vi "Parse RMC Sentence.vi"(8 "error in (no error)":errorcluster, 11 "RMC sentence":string) -> (0 "error out":errorcluster, 3 "RMC data":T1 {"type of fix"."mode" items=["Simulator", "Not Valid", "Estimated", "Differential", "Autonomous"]; "status"."value" items=["Void", "Active"]; "time of fix"."time (UTC)" format=" %^<%.3X\n%x>T"})   [LabVIEW 2017, in "NMEA API.lvlib"]
doc: "Returns data contained in a particular type of NMEA sentence. The input sentence you specify must include valid NMEA formatting and end with a carriage return and line feed, or \\r\\n. You must manually select the polymorphic instance to use."
uses:
  <vilib>/robotics/Protocols/NMEA/NMEA API.lvlib
  <vilib>/robotics/Protocols/NMEA/typedefs/RMC Data.ctl
  <vilib>/Utility/miscctls.llb/LVDateTimeRec.ctl
  <vilib>/robotics/Utilities/NI_Robotics Utilities.lvlib
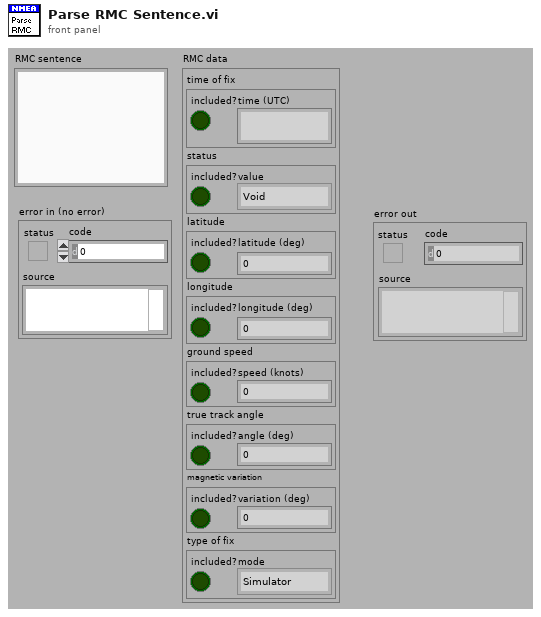
[diagram p1: front panel]
types:
  T1 = typedef "NMEA API.lvlib/RMC Data.ctl" = cluster{"time of fix":cluster{"included?":bool, "time (UTC)":timestamp}, "status":cluster{"included?":bool, "value":u16}, "latitude":cluster{"included?":bool, "latitude (deg)":dbl}, "longitude":cluster{"included?":bool, "longitude (deg)":dbl}, "ground speed":cluster{"included?":bool, "speed (knots)":dbl}, "true track angle":cluster{"included?":bool, "angle (deg)":dbl}, "magnetic variation":cluster{"included?":bool, "variation (deg)":dbl}, "type of fix":cluster{"included?":bool, "mode":u16}}
  T2 = typedef "LVDateTimeRec.ctl" = cluster{"fractional second":dbl, "second":i32, "minute":i32, "hour":i32, "day of month":i32, "month":i32, "year":i32, "day of week":i32, "day of year":i32, "DST":i32}
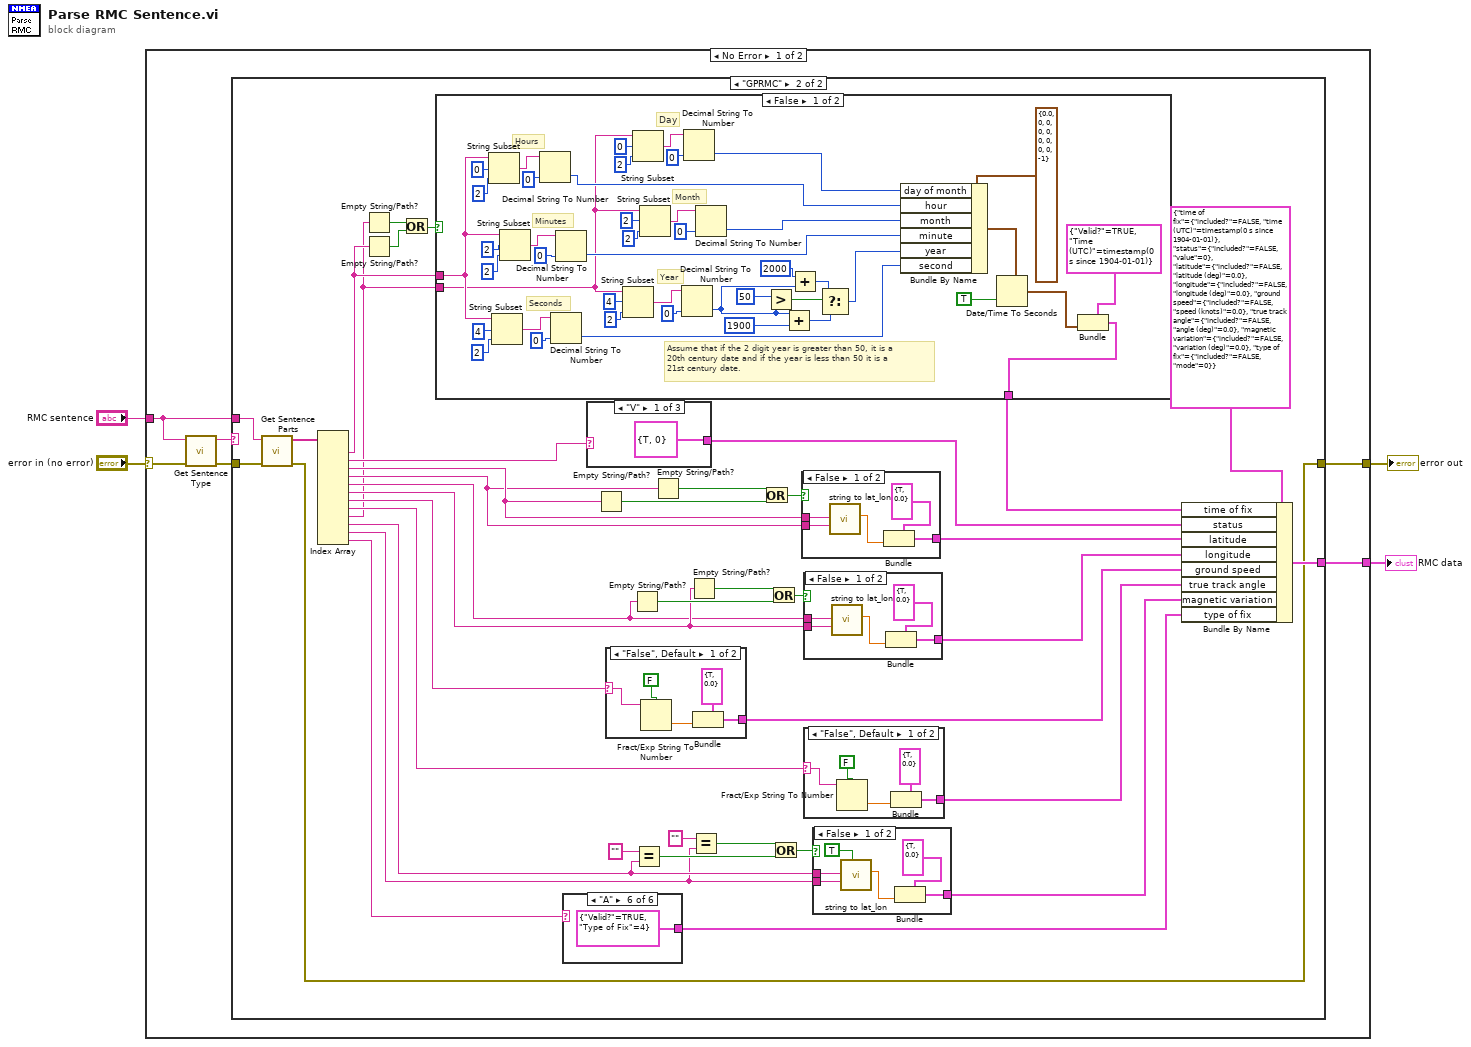
[diagram p0: block diagram]
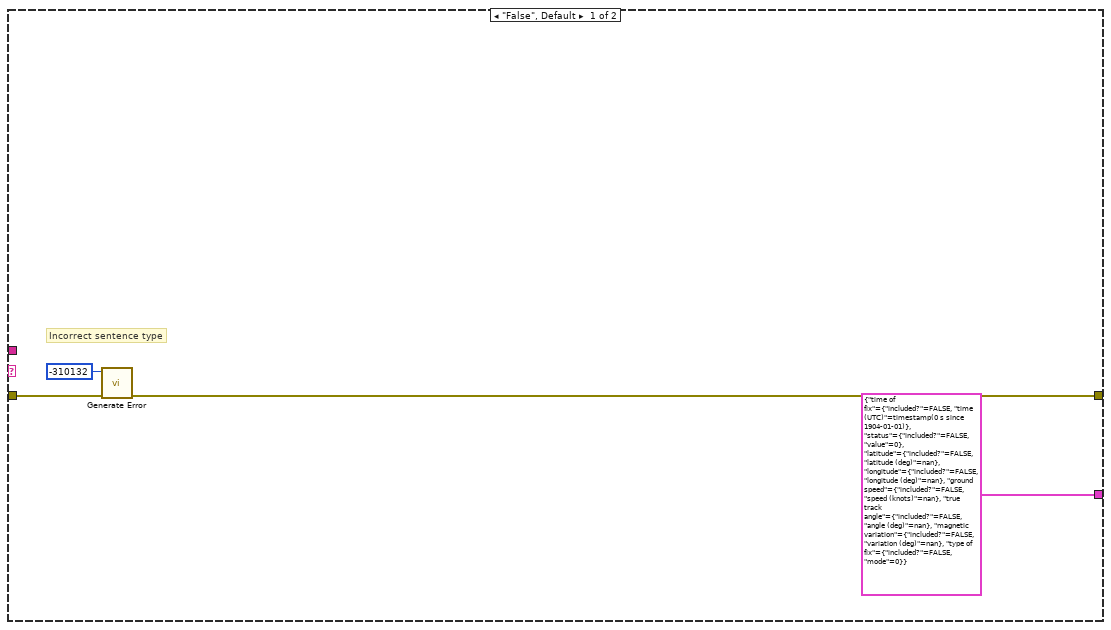
[diagram p2: hidden frame]
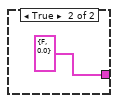
[diagram p3: hidden frame]
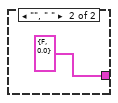
[diagram p4: hidden frame]
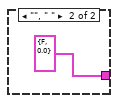
[diagram p5: hidden frame]
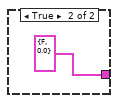
[diagram p6: hidden frame]
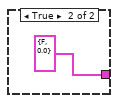
[diagram p7: hidden frame]
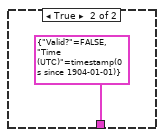
[diagram p8: hidden frame]
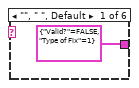
[diagram p9: hidden frame]
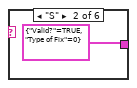
[diagram p10: hidden frame]
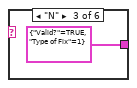
[diagram p11: hidden frame]
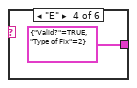
[diagram p12: hidden frame]
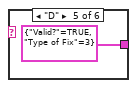
[diagram p13: hidden frame]
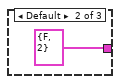
[diagram p14: hidden frame]
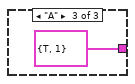
[diagram p15: hidden frame]
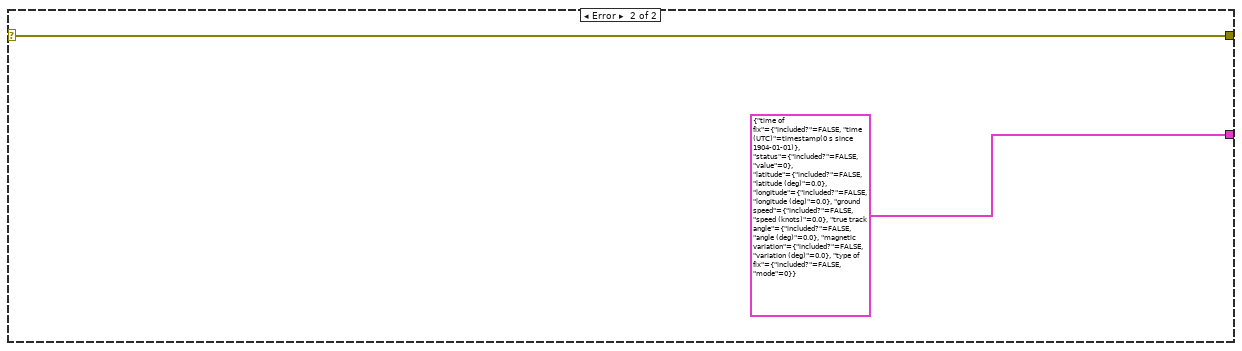
[diagram p16: hidden frame]
diagram:
  n1 = case shown="No Error" "error in (no error)" {
    selector: "error in (no error)" -> [w8 w142]
    tunnel: [w9 w142] -> w2
    tunnel: [w10 T1 {"time of fix"={"included?"=FALSE, "time (UTC)"=timestamp(0 s since 1904-01-01)}, "status"={"included?"=FALSE, "value"=0}, "latitude"={"included?"=FALSE, "latitude (deg)"=0.0}, "longitude"={"included?"=FALSE, "longitude (deg)"=0.0}, "ground speed"={"included?"=FALSE, "speed (knots)"=0.0}, "true track angle"={"included?"=FALSE, "angle (deg)"=0.0}, "magnetic variation"={"included?"=FALSE, "variation (deg)"=0.0}, "type of fix"={"included?"=FALSE, "mode"=0}} ("RMC Data")] -> w1
    tunnel: "RMC sentence" -> [w6 _]
    frame No Error {
      n2 = call <vilib>:"Get Sentence Type.vi"("error in (no error)"=w8, "sentence"=w6) -> ("error out"=w7:errorcluster, "sentence type"=w5:string)  [unwired: 1 in, 7 out]
      n3 = case shown="\"GPRMC\"" w5 {
        tunnel: w6 -> [_ w18]
        tunnel: w7 -> [w12 w54]
        tunnel: [T1 {"time of fix"={"included?"=FALSE, "time (UTC)"=timestamp(0 s since 1904-01-01)}, "status"={"included?"=FALSE, "value"=0}, "latitude"={"included?"=FALSE, "latitude (deg)"=nan}, "longitude"={"included?"=FALSE, "longitude (deg)"=nan}, "ground speed"={"included?"=FALSE, "speed (knots)"=nan}, "true track angle"={"included?"=FALSE, "angle (deg)"=nan}, "magnetic variation"={"included?"=FALSE, "variation (deg)"=nan}, "type of fix"={"included?"=FALSE, "mode"=0}} ("RMC Data") w53] -> w10
        tunnel: [w11 w16] -> w9
        frame "False", Default {
          # "Incorrect sentence type"
          n4 = call <vilib>:"Generate Error.vi"("error in (no error)"=w12, "code"=-310132) -> ("error out"=w11:errorcluster)  [unwired: 9 in]
        }
        frame "GPRMC" {
          n5 = call <vilib>:"Get Sentence Parts.vi"("error in (no error)"=w54, "sentence"=w18) -> ("error out"=w16:errorcluster, "sentence data"=w17:string[])  [unwired: 1 in, 7 out]
          n6 = Index Array(array=w17) -> (element #1=w46:string, element #2=w51:string, element #3=w42:string, element #4=w41:string, element #5=w32:string, element #6=w33:string, element #7=w31:string, element #8=w29:string, element #9=w15:string, element #10=w22:string, element #11=w21:string, element #12=w50:string)  [unwired: 12 in]
          n7 = Empty String/Path?(string/path=w15) -> (empty?=w48:bool)
          n8 = Empty String/Path?(string/path=w46) -> (empty?=w49:bool)
          n9 = Or(x=w48, y=w49) -> (x .or. y?=w47:bool)
          n10 = case shown="False" w47 {
            tunnel: [w95 cluster{"Valid?":bool, "Time (UTC)":timestamp} {"Valid?"=FALSE, "Time (UTC)"=timestamp(0 s since 1904-01-01)} ("Time of Fix")] -> w45
            tunnel: w46 -> [w99 _]
            tunnel: w15 -> [w98 _]
            frame False {
              # "Assume that if the 2 digit year is greater than 50, it is a\n20th century date and if the year is less than 50 it is a \n21st century date."
              # "Year"
              # "Month"
              # "Day"
              # "Seconds"
              # "Minutes"
              # "Hours"
              n11 = String Subset(string=w99, offset (0)=0 ("length (rest)"), length (rest)=2 ("length (rest)")) -> (substring=w123:string)
              n12 = String Subset(string=w99, offset (0)=4 ("length (rest)"), length (rest)=2 ("length (rest)")) -> (substring=w127:string)
              n13 = String Subset(string=w99, offset (0)=2 ("length (rest)"), length (rest)=2 ("length (rest)")) -> (substring=w124:string)
              n14 = Decimal String To Number(string=w123, default (0L)=0 ("default (0 DBL)")) -> (number=w105:i32)  [unwired: 2 out]
              n15 = Decimal String To Number(string=w127, default (0L)=0 ("default (0 DBL)")) -> (number=w102:i32)  [unwired: 2 out]
              n16 = Decimal String To Number(string=w124, default (0L)=0 ("default (0 DBL)")) -> (number=w103:i32)  [unwired: 2 out]
              n17 = String Subset(string=w98, offset (0)=4 ("length (rest)"), length (rest)=2 ("length (rest)")) -> (substring=w116:string)
              n18 = String Subset(string=w98, offset (0)=0 ("length (rest)"), length (rest)=2 ("length (rest)")) -> (substring=w120:string)
              n19 = String Subset(string=w98, offset (0)=2 ("length (rest)"), length (rest)=2 ("length (rest)")) -> (substring=w119:string)
              n20 = Decimal String To Number(string=w116, default (0L)=0 ("default (0 DBL)")) -> (number=w89:i32)  [unwired: 2 out]
              n21 = Decimal String To Number(string=w120, default (0L)=0 ("default (0 DBL)")) -> (number=w106:i32)  [unwired: 2 out]
              n22 = Decimal String To Number(string=w119, default (0L)=0 ("default (0 DBL)")) -> (number=w104:i32)  [unwired: 2 out]
              n23 = Greater?(x=50, y=w89) -> (0:w93:bool)
              n24 = Add(x=w89, y=1900) -> (x+y=w91:i32)
              n25 = Add(x=2000, y=w89) -> (x+y=w90:i32)
              n26 = Select(t=w90, s=w93, f=w91) -> (s? t:f=w87:i32)
              n27 = Bundle By Name(cluster=T2 {"fractional second"=0.0, "second"=0, "minute"=0, "hour"=0, "day of month"=0, "month"=0, "year"=0, "day of week"=0, "day of year"=0, "DST"=-1} ("date time rec"), "day of month"=w106, "hour"=w105, "month"=w104, "minute"=w103, "year"=w87, "second"=w102) -> (w101:T2)
              n28 = Date/Time To Seconds(1:TRUE, 2:w101) -> (0:w96:timestamp)
              n29 = Bundle(cluster=cluster{"Valid?":bool, "Time (UTC)":timestamp} {"Valid?"=TRUE, "Time (UTC)"=timestamp(0 s since 1904-01-01)} ("Time of Fix"), "Time (UTC)"=w96) -> (w95:cluster{"Valid?":bool, "Time (UTC)":timestamp})  [unwired: 1 out]
            }
            frame True {
            }
          }
          n30 = case shown="\"A\"" w50 {
            tunnel: [cluster{"Valid?":bool, "Type of Fix":u16} {"Valid?"=FALSE, "Type of Fix"=1} ("Type of Fix") cluster{"Valid?":bool, "Type of Fix":u16} {"Valid?"=TRUE, "Type of Fix"=0} ("Type of Fix") cluster{"Valid?":bool, "Type of Fix":u16} {"Valid?"=TRUE, "Type of Fix"=1} ("Type of Fix") cluster{"Valid?":bool, "Type of Fix":u16} {"Valid?"=TRUE, "Type of Fix"=2} ("Type of Fix") cluster{"Valid?":bool, "Type of Fix":u16} {"Valid?"=TRUE, "Type of Fix"=3} ("Type of Fix") cluster{"Valid?":bool, "Type of Fix":u16} {"Valid?"=TRUE, "Type of Fix"=4} ("Type of Fix")] -> w19
            frame "", " ", Default {
            }
            frame "S" {
            }
            frame "N" {
            }
            frame "E" {
            }
            frame "D" {
            }
            frame "A" {
            }
          }
          n31 = case shown="\"V\"" w51 {
            tunnel: [cluster{"Valid?":bool, "Status":u16} {"Valid?"=TRUE, "Status"=0} ("Status") cluster{"Valid?":bool, "Status":u16} {"Valid?"=FALSE, "Status"=2} ("Status") cluster{"Valid?":bool, "Status":u16} {"Valid?"=TRUE, "Status"=1} ("Status")] -> w40
            frame "V" {
            }
            frame Default {
            }
            frame "A" {
            }
          }
          n32 = Empty String/Path?(string/path=w42) -> (empty?=w43:bool)
          n33 = case shown="\"False\", Default" w31 {
            selector: w31 -> [w72 _]
            tunnel: [w69 cluster{"Valid?":bool, "Speed (Knots)":dbl} {"Valid?"=FALSE, "Speed (Knots)"=0.0} ("Ground Speed")] -> w30
            frame "False", Default {
              n34 = Fract/Exp String To Number(use system decimal point (T)=FALSE, string=w72) -> (number=w70:dbl)  [unwired: 3 out]
              n35 = Bundle(cluster=cluster{"Valid?":bool, "Speed (Knots)":dbl} {"Valid?"=TRUE, "Speed (Knots)"=0.0} ("Ground Speed"), "Speed (Knots)"=w70) -> (w69:cluster{"Valid?":bool, "Speed (Knots)":dbl})  [unwired: 1 out]
            }
            frame "", " " {
            }
          }
          n36 = Empty String/Path?(string/path=w32) -> (empty?=w36:bool)
          n37 = Equal?(x="", y=w22) -> (x = y?=w24:bool)
          n38 = Empty String/Path?(string/path=w41) -> (empty?=w44:bool)
          n39 = Empty String/Path?(string/path=w33) -> (empty?=w35:bool)
          n40 = Equal?(x="", y=w21) -> (x = y?=w25:bool)
          n41 = Or(x=w44, y=w43) -> (x .or. y?=w39:bool)
          n42 = Or(x=w35, y=w36) -> (x .or. y?=w34:bool)
          n43 = Or(x=w25, y=w24) -> (x .or. y?=w23:bool)
          n44 = case shown="False" w39 {
            tunnel: w42 -> [w84 _]
            tunnel: w41 -> [w83 _]
            tunnel: [w80 cluster{"Valid?":bool, "Latitude (Deg)":dbl} {"Valid?"=FALSE, "Latitude (Deg)"=0.0} ("Latitude")] -> w38
            frame False {
              n45 = call <vilib>:"string to lat_lon.vi"("direction string"=w83, "numeric string for lat/lon"=w84) -> ("composite value"=w82:dbl)  [unwired: 1 in, 8 out]
              n46 = Bundle(cluster=cluster{"Valid?":bool, "Latitude (Deg)":dbl} {"Valid?"=TRUE, "Latitude (Deg)"=0.0} ("Latitude"), "Latitude (Deg)"=w82) -> (w80:cluster{"Valid?":bool, "Latitude (Deg)":dbl})  [unwired: 1 out]
            }
            frame True {
            }
          }
          n47 = case shown="False" w34 {
            tunnel: w32 -> [w78 _]
            tunnel: w33 -> [w77 _]
            tunnel: [w74 cluster{"Valid?":bool, "Latitude (Deg)":dbl} {"Valid?"=FALSE, "Latitude (Deg)"=0.0} ("Latitude")] -> w37
            frame False {
              n48 = call <vilib>:"string to lat_lon.vi"("direction string"=w77, "numeric string for lat/lon"=w78) -> ("composite value"=w76:dbl)  [unwired: 1 in, 8 out]
              n49 = Bundle(cluster=cluster{"Valid?":bool, "Latitude (Deg)":dbl} {"Valid?"=TRUE, "Latitude (Deg)"=0.0} ("Latitude"), "Latitude (Deg)"=w76) -> (w74:cluster{"Valid?":bool, "Latitude (Deg)":dbl})  [unwired: 1 out]
            }
            frame True {
            }
          }
          n50 = case shown="\"False\", Default" w29 {
            selector: w29 -> [w66 _]
            tunnel: [w63 cluster{"Valid?":bool, "Speed (Knots)":dbl} {"Valid?"=FALSE, "Speed (Knots)"=0.0} ("Ground Speed")] -> w28
            frame "False", Default {
              n51 = Fract/Exp String To Number(use system decimal point (T)=FALSE, string=w66) -> (number=w64:dbl)  [unwired: 3 out]
              n52 = Bundle(cluster=cluster{"Valid?":bool, "Speed (Knots)":dbl} {"Valid?"=TRUE, "Speed (Knots)"=0.0} ("Ground Speed"), "Speed (Knots)"=w64) -> (w63:cluster{"Valid?":bool, "Speed (Knots)":dbl})  [unwired: 1 out]
            }
            frame "", " " {
            }
          }
          n53 = case shown="False" w23 {
            tunnel: w22 -> [w60 _]
            tunnel: w21 -> [w59 _]
            tunnel: [w56 cluster{"Valid?":bool, "Latitude (Deg)":dbl} {"Valid?"=FALSE, "Latitude (Deg)"=0.0} ("Latitude")] -> w20
            frame False {
              n54 = call <vilib>:"string to lat_lon.vi"("magnetic variation?"=TRUE ("Magnetic Variation?"), "direction string"=w59, "numeric string for lat/lon"=w60) -> ("composite value"=w58:dbl)  [unwired: 8 out]
              n55 = Bundle(cluster=cluster{"Valid?":bool, "Latitude (Deg)":dbl} {"Valid?"=TRUE, "Latitude (Deg)"=0.0} ("Latitude"), "Latitude (Deg)"=w58) -> (w56:cluster{"Valid?":bool, "Latitude (Deg)":dbl})  [unwired: 1 out]
            }
            frame True {
            }
          }
          n56 = Bundle By Name(cluster=T1 {"time of fix"={"included?"=FALSE, "time (UTC)"=timestamp(0 s since 1904-01-01)}, "status"={"included?"=FALSE, "value"=0}, "latitude"={"included?"=FALSE, "latitude (deg)"=0.0}, "longitude"={"included?"=FALSE, "longitude (deg)"=0.0}, "ground speed"={"included?"=FALSE, "speed (knots)"=0.0}, "true track angle"={"included?"=FALSE, "angle (deg)"=0.0}, "magnetic variation"={"included?"=FALSE, "variation (deg)"=0.0}, "type of fix"={"included?"=FALSE, "mode"=0}} ("RMC Data"), "time of fix"=w45, "status"=w40, "latitude"=w38, "longitude"=w37, "ground speed"=w30, "true track angle"=w28, "magnetic variation"=w20, "type of fix"=w19) -> (w53:T1)
        }
      }
    }
    frame Error {
    }
  }
  "error out" <- w2
  "RMC data" <- w1
